vi "SeriesStringGenerator.vi"(1 "Array":i32[](array[numeric])) -> (0 "series string":string)   [LabVIEW 2024]
uses:
  4113e1fe-fd04-4a93-bd5d-83474d822903.vi
  <userlib>/_OpenG.lib/string/string.llb/openg_string.lvlib
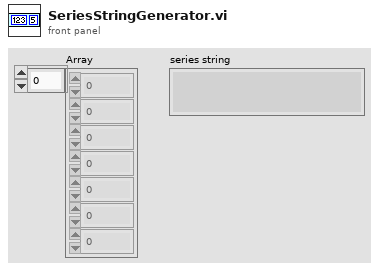
[diagram p1: front panel]
types:
  T1 = enum16{"Init", "Process Element", "End of Range", "End"}
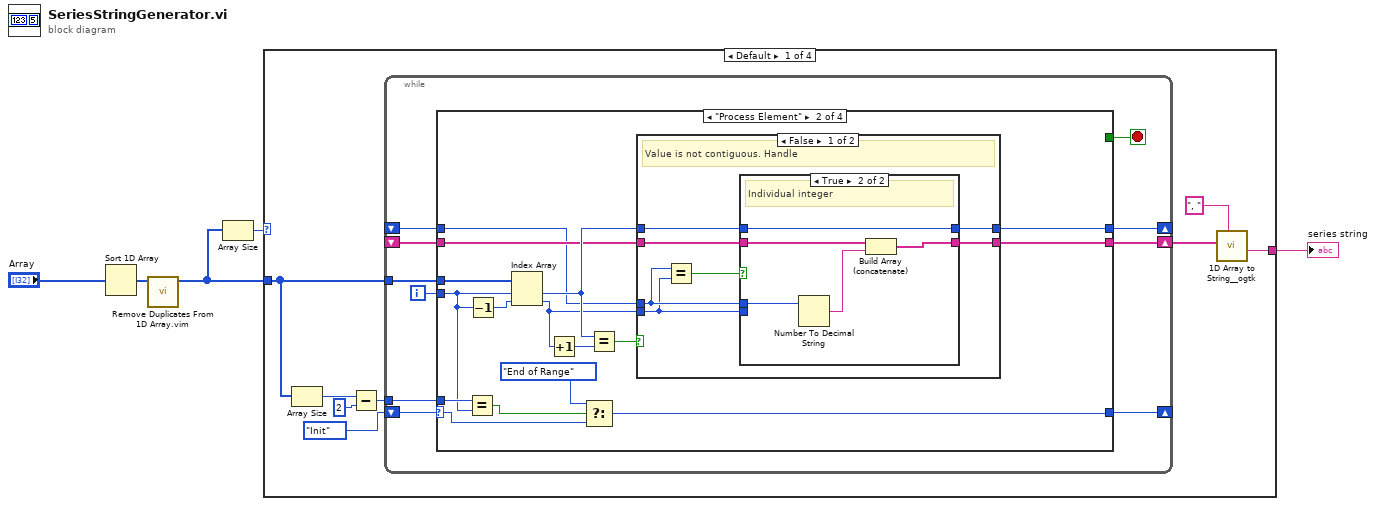
[diagram p0: block diagram]
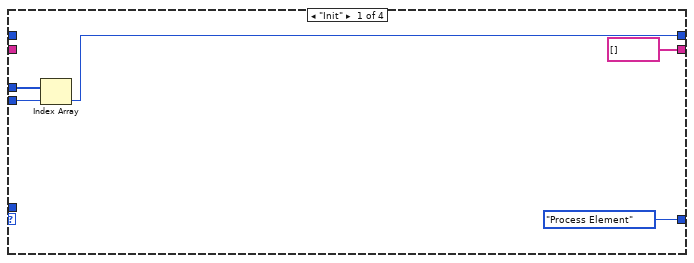
[diagram p2: hidden frame]
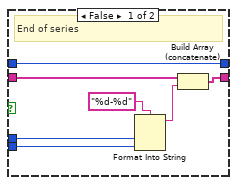
[diagram p3: hidden frame]
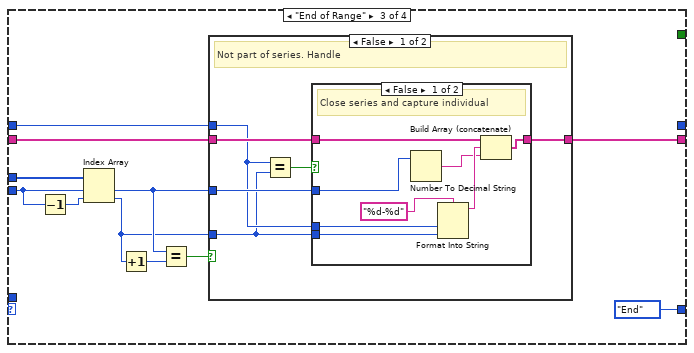
[diagram p5: hidden frame]
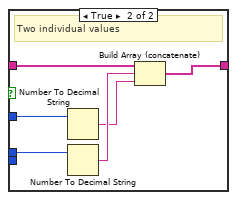
[diagram p6: hidden frame]
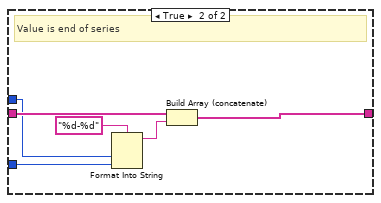
[diagram p7: hidden frame]
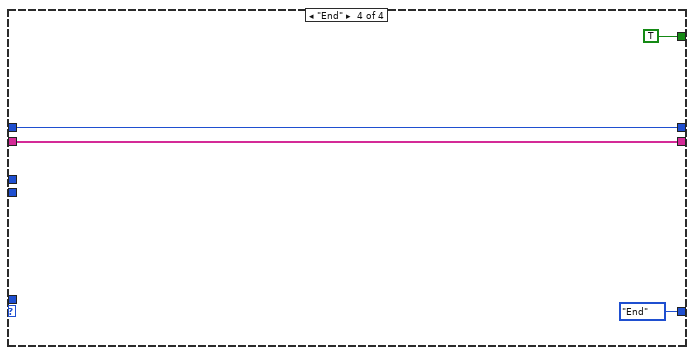
[diagram p8: hidden frame]
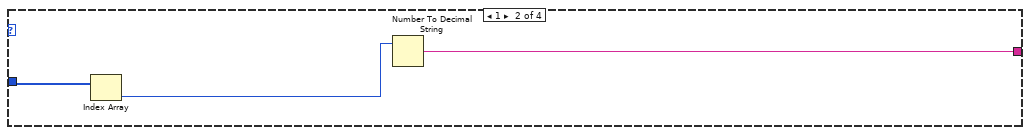
[diagram p9: hidden frame]
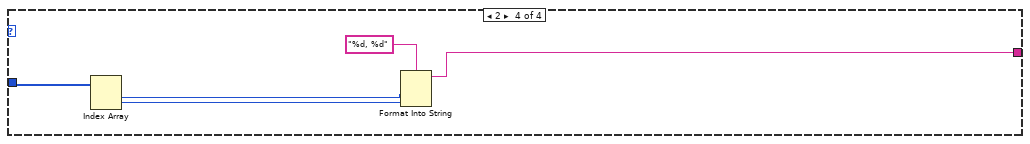
[diagram p11: hidden frame]
diagram:
  n1 = Sort 1D Array(array="Array") -> (sorted array=w2:i32[])
  n2 = call "Remove Duplicates From 1D Array.vim"("array"=w2) -> ("array with duplicates removed"=w1:i32[])  [unwired: 10 in]
  n3 = Array Size(array=w1) -> (size(s)=w4:i32)
  n4 = case shown="Default" w4 {
    tunnel: w1 -> [w6 w109 _ w114]
    tunnel: [w7 w107 _ w113] -> w5
    frame Default {
      n5 = Array Size(array=w6) -> (size(s)=w12:i32)
      n6 = Subtract(x=w12, y=2) -> (x-y=w10:i32)
      n7 = while {
        tunnel: w6 -> [w20]
        shift-right: [w22] -> _
        shift-left: T1."Init" -> [w23]
        shift-right: [w21] -> w9
        shift-left: _ -> [w17]
        shift-right: [w18] -> _
        shift-left: _ -> [w14]
        tunnel: w10 -> [w16]
        i -> [w19]
        stop <- w15 stop-if-true
        n8 = case shown="\"Process Element\"" w23 {
          selector: w23 -> [_ w33 _ _]
          tunnel: [T1."Process Element" w32 T1."End" ("t") T1."End" ("t")] -> w22
          tunnel: [string[] [] w38 w71 w105] -> w21
          tunnel: w20 -> [w26 w44 w76 _]
          tunnel: w19 -> [w25 w35 w69 _]
          tunnel: [w24 w41 _ w103] -> w18
          tunnel: w17 -> [_ w39 w72 w105]
          tunnel: w14 -> [_ w30 w68 w103]
          tunnel: w16 -> [_ w36 _ _]
          tunnel: [_ _ _ TRUE] -> w15
          frame "Init" {
            n9 = Index Array(array=w26, index=w25) -> (element=w24:i32)
          }
          frame "Process Element" {
            n10 = Equal?(x=w36, y=w35) -> (x = y?=w34:bool)
            n11 = Decrement(x=w35) -> (x-1=w37:i32)
            n12 = Index Array(array=w44, index #1=w35, index #2=w37) -> (element #1=w40:i32, element #2=w29:i32)
            n13 = Increment(x=w29) -> (x+1=w43:i32)
            n14 = Select(t=T1."End of Range", s=w34, f=w33) -> (s? t:f=w32:T1)
            n15 = Equal?(x=w40, y=w43) -> (x = y?=w42:bool)
            n16 = case shown="False" w42 {
              tunnel: [w47 w64] -> w41
              tunnel: w40 -> [w48 _]
              tunnel: w30 -> [w46 w64]
              tunnel: w39 -> [w50 w65]
              tunnel: [w49 w65] -> w38
              tunnel: w29 -> [w45 _]
              frame False {
                # "Value is not contiguous. Handle"
                n17 = Equal?(x=w46, y=w45) -> (x = y?=w51:bool)
                n18 = case shown="True" w51 {
                  tunnel: w46 -> [w57 w63]
                  tunnel: w50 -> [w56 w61]
                  tunnel: [w54 w60] -> w49
                  tunnel: w48 -> [w52 w59]
                  tunnel: w45 -> [w53 _]
                  tunnel: [w52 w59] -> w47
                  frame False {
                    # "End of series"
                    n19 = Format Into String(format string="%d-%d", w57, w53) -> (resulting string=w55:string)  [unwired: 2 in, 1 out]
                    n20 = Build Array (concatenate)(w56, w55) -> (w54:string[])
                  }
                  frame True {
                    # "Individual integer"
                    n21 = Number To Decimal String(number=w63) -> (decimal integer string=w62:string)  [unwired: 1 in]
                    n22 = Build Array (concatenate)(w61, w62) -> (w60:string[])
                  }
                }
              }
              frame True {
                # "Value is contiguous.  Continue"
              }
            }
          }
          frame "End of Range" {
            n23 = Decrement(x=w69) -> (x-1=w70:i32)
            n24 = Index Array(array=w76, index #1=w69, index #2=w70) -> (element #1=w73:i32, element #2=w67:i32)
            n25 = Increment(x=w67) -> (x+1=w75:i32)
            n26 = Equal?(x=w73, y=w75) -> (x = y?=w74:bool)
            n27 = case shown="False" w74 {
              tunnel: w73 -> [w79 w97]
              tunnel: w68 -> [w78 w98]
              tunnel: w72 -> [w81 w100]
              tunnel: [w80 w99] -> w71
              tunnel: w67 -> [w77 _]
              frame False {
                # "Not part of series. Handle"
                n28 = Equal?(x=w78, y=w77) -> (x = y?=w82:bool)
                n29 = case shown="False" w82 {
                  tunnel: w78 -> [w89 w96]
                  tunnel: w81 -> [w88 w94]
                  tunnel: [w86 w93] -> w80
                  tunnel: w79 -> [w84 w92]
                  tunnel: w77 -> [w85 _]
                  frame False {
                    # "Close series and capture individual"
                    n30 = Number To Decimal String(number=w84) -> (decimal integer string=w83:string)  [unwired: 1 in]
                    n31 = Format Into String(format string="%d-%d", w89, w85) -> (resulting string=w87:string)  [unwired: 2 in, 1 out]
                    n32 = Build Array (concatenate)(w88, w87, w83) -> (w86:string[])
                  }
                  frame True {
                    # "Two individual values"
                    n33 = Number To Decimal String(number=w92) -> (decimal integer string=w91:string)  [unwired: 1 in]
                    n34 = Number To Decimal String(number=w96) -> (decimal integer string=w95:string)  [unwired: 1 in]
                    n35 = Build Array (concatenate)(w94, w95, w91) -> (w93:string[])
                  }
                }
              }
              frame True {
                # "Value is end of series"
                n36 = Format Into String(format string="%d-%d", w98, w97) -> (resulting string=w101:string)  [unwired: 2 in, 1 out]
                n37 = Build Array (concatenate)(w100, w101) -> (w99:string[])
              }
            }
          }
          frame "End" {
          }
        }
      }
      n38 = call <userlib>:"1D Array to String__ogtk.vi"("delimiter (Tab)"=", ", "Array of Strings"=w9) -> ("delimited string"=w7:string)  [unwired: 9 in]
    }
    frame 1 {
      n39 = Index Array(array=w109) -> (element=w108:i32)  [unwired: 1 in]
      n40 = Number To Decimal String(number=w108) -> (decimal integer string=w107:string)  [unwired: 1 in]
    }
    frame 0 {
    }
    frame 2 {
      n41 = Index Array(array=w114) -> (element #1=w111:i32, element #2=w110:i32)  [unwired: 2 in]
      n42 = Format Into String(format string="%d, %d", w111, w110) -> (resulting string=w113:string)  [unwired: 2 in, 1 out]
    }
  }
  "series string" <- w5
